vi "failures lverror to failure.vi"(8 "error in":errorcluster) -> (0 "failure":T1 {"code" format="%.0x"})   [LabVIEW 2013]
uses:
  failure.ctl
  <vilib>/Utility/error.llb/TagReturnType.ctl
  const sourcename.vi
  const messagename.vi
  failure.lvlib
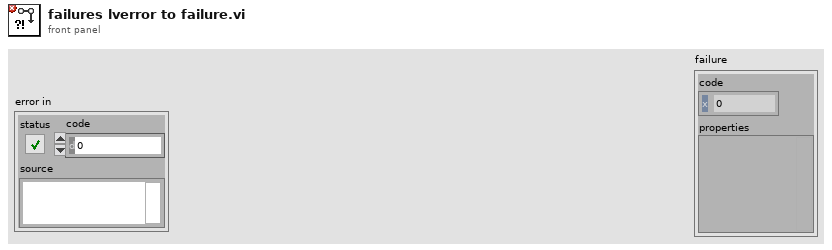
[diagram p1: front panel]
types:
  T1 = typedef "failure.lvlib/failure.ctl" = cluster{"code":i32, "properties":variant}
  T2 = typedef "TagReturnType.ctl" = enum16{"No Tag", "<err>", "<append>"}
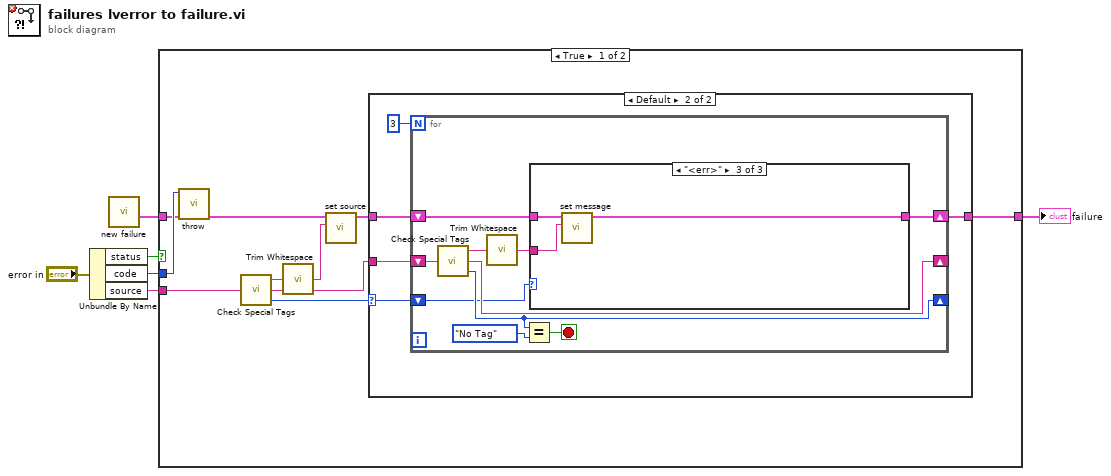
[diagram p0: block diagram]
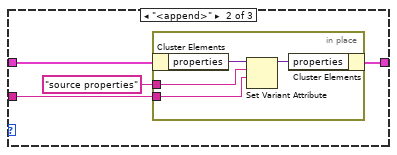
[diagram p4: hidden frame]
diagram:
  n1 = Unbundle By Name("error in") -> ("status"=w1:bool, "code"=w4:i32, "source"=w5:string)
  n2 = call "new failure.vi"() -> ("failure"=w2:T1)  [unwired: 11 in]
  n3 = case shown="True" w1 {
    tunnel: [w14 w45] -> w6
    tunnel: w5 -> [w16 _]
    tunnel: w4 -> [w13 _]
    tunnel: w2 -> [w12 w45]
    frame True {
      n4 = call "throw.vi"("failure in"=w12, "code"=w13) -> ("failure"=w15:T1)  [unwired: 9 in]
      n5 = call <vilib>:"Check Special Tags.vi"("source"=w16) -> ("Before Tag (source)"=w11:string, "After Tag (special data)"=w9:string, "Tag Found?"=w8:T2)
      n6 = call <vilib>:"Trim Whitespace.vi"("string"=w11) -> ("trimmed string"=w7:string)  [unwired: 1 in]
      n7 = call "set source.vi"("source"=w7, "failure in"=w15) -> ("failure out"=w10:T1)  [unwired: 9 in]
      n8 = case shown="Default" w8 {
        selector: w8 -> [_ w19]
        tunnel: w10 -> [w17 w22]
        tunnel: [w17 w21] -> w14
        tunnel: w9 -> [_ w20]
        frame "No Tag" {
        }
        frame Default {
          n9 = for {
            N: 3 -> [_]
            shift-right: [w25] -> w21
            shift-left: w22 -> [w24]
            shift-right: [w31] -> _
            shift-left: w20 -> [w32]
            shift-right: [w30] -> _
            shift-left: w19 -> [w27]
            stop <- w28 stop-if-true
            n10 = call <vilib>:"Check Special Tags.vi"("source"=w32) -> ("Before Tag (source)"=w26:string, "After Tag (special data)"=w31:string, "Tag Found?"=w30:T2)
            n11 = call <vilib>:"Trim Whitespace.vi"("string"=w26) -> ("trimmed string"=w23:string)  [unwired: 1 in]
            n12 = Equal?(x=w30, y=TagReturnType."No Tag") -> (x = y?=w28:bool)
            n13 = case shown="\"<err>\"" w27 {
              tunnel: w23 -> [_ w34 w42]
              tunnel: [w33 w36 w43] -> w25
              tunnel: w24 -> [w33 w37 w44]
              frame "No Tag" {
              }
              frame "<append>" {
                n14 = in-place {
                  in-place-border: "source properties" ("label") -> [w39]
                  in-place-border: w34 -> [w38]
                  n15 = in-place-cluster #1(w37) -> ("properties"=w41:variant)
                  n16 = Set Variant Attribute(Variant=w41, name=w39, value=w38) -> (Variant out=w40:variant)  [unwired: 1 in, 2 out]
                  n17 = in-place-cluster #1("properties"=w40) -> (w36:T1)
                }
              }
              frame "<err>" {
                n18 = call "set message.vi"("message"=w42, "failure in"=w44) -> ("failure out"=w43:T1)  [unwired: 9 in]
              }
            }
          }
        }
      }
    }
    frame False {
    }
  }
  "failure" <- w6
